vi "test.vi"() -> ()   [LabVIEW 2018]
uses:
  <vilib>/imath/engines/lvmath/Plug In/_Char/NIMS_CH_character datatype.ctl
  <vilib>/imath/engines/lvmath2/RunTimeEngine/Managers/WorkSpace/UID Generator.vi
  <vilib>/imath/engines/lvmath2/RunTimeEngine/RunTimeType/NIMS_RunTimeType_From StrictType (excl LVString).vi
  <instcachedir>/0/NIMS_RunTimeType_From StrictType (excl LVString)_E7E34A65C99947108168652BAD14964D.lvgen/NIMS_RunTimeType_From StrictType (excl LVString)_E7E34A65C99947108168652BAD14964D_000.vi
  <vilib>/imath/engines/lvmath2/RunTimeEngine/LocalVariableDefStatement/MC_LocalVariableDefStatement_Display.vi
  <vilib>/imath/engines/lvmath/Plug In/_Char/NIMS_CH_Character RV to String.vi
  Documents/LabVIEW Data/MathScriptVIs/MCStatic_40275148932_9249425576578f2cef5e9c0da6b682b6.vi
  <vilib>/imath/engines/lvmath2/RunTimeEngine/BuiltInFunctions/ode_rk23/NIMS_[RV,RM]=ode_rk23.vi
  <vilib>/imathl/engines/lvmath/Functions/Error Handling/Create Error.vi
  <vilib>/imath/engines/lvmath2/RunTimeEngine/Managers/SymbolTable/Clear UID.vi
  <vilib>/imath/engines/lvmath2/RunTimeEngine/NodeEndStatement/NIMS_NodeEndStatement_Output.vi
  <instcachedir>/0/NIMS_NodeEndStatement_Output_53EC0D466D134D7ABD903AC30B43404B.lvgen/NIMS_NodeEndStatement_Output_53EC0D466D134D7ABD903AC30B43404B_002.vi
  <instcachedir>/0/NIMS_NodeEndStatement_Output_53EC0D466D134D7ABD903AC30B43404B.lvgen/NIMS_NodeEndStatement_Output_53EC0D466D134D7ABD903AC30B43404B_001.vi
  <vilib>/imath/engines/lvmath2/RunTimeEngine/ErrorHandling/NIMS_Finalize Error.vi
  Documents/LabVIEW Data/ode_lv.m
  <vilib>/imath/engines/lvmath2/RunTimeEngine/Managers/SymbolTable/NIMS_WorkSpace.lvlib
panel:
  out "s":dbl[][](array[numeric])
  out "y":dbl
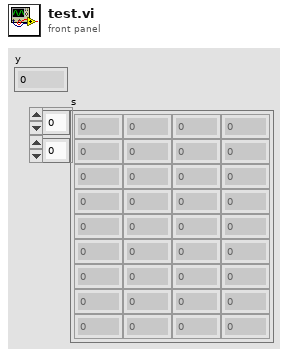
[diagram p1: front panel]
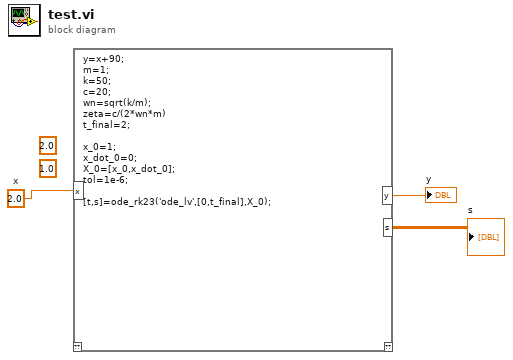
[diagram p0: block diagram]
diagram:
  (unwired) 2.0 ("Tg")
  (unwired) 1.0 ("Ta")
  w3 = 2.0  # x
  n1 = mathscript code="y=x+90;\nm=1;\nk=50;\nc=20;\nwn=sqrt(k/m);\nzeta=c/(2*wn*m)\nt_final=2;\n\nx_0=1;\nx_dot_0=0;\nX_0=[x_0,x_dot_0];\ntol=1e-6;\n\n[t,s]=ode_rk23('ode_lv',[0,t_final],X_0);"("x"=w3) -> ("y"=→"y":dbl, "s"=→"s":dbl[][])  [unwired: 1 in, 1 out]
